vi "LIDAR V3.1 FPGA Main.vi"() -> ()   [LabVIEW 2013]
uses:
  Controls/FPGA Nain State.ctl
  <vilib>/Platform/TimedLoop/XDataNode/timing_clust.ctl
  <vilib>/Platform/TimedLoop/XDataNode/nitl_modes.ctl
  <vilib>/Platform/TimedLoop/XDataNode/wakeup.ctl
  Controls/Algorithm State.ctl
  <vilib>/rvi/Emulation/niFpgaSctlEmulationGetInTimedLoop.vi
  <vilib>/rvi/Emulation/niFpgaEmulationReportErrorSimple.vi
  <vilib>/rvi/Emulation/niFpgaGetClockAttributes.vi
  <vilib>/rvi/Emulation/niFpgaCriticalErrorInLSC.vi
  <vilib>/rvi/FIFO/Fifo_Resource/nirvififoEmulationReadFpgaImpl.vi
  <vilib>/rvi/DataTransferAndStorage/Container/Common/niFpgaContainerGetUniqueNameForEmu.vi
  <vilib>/rvi/FIFO/Fifo_Resource/nirvififoEmulationWriteFpgaImpl.vi
  <vilib>/rvi/interface/RandomDataEmulation/nirviRandomDataFPGAFIFO.vi
  <vilib>/rvi/interface/RandomDataEmulation/niFpgaRandomDataHandleErrors.vi
  <vilib>/rvi/eio/common/nirviEmuTemplateMethod_errors.vi
  <vilib>/rvi/Memory/Memory_Emulation/nirvimemoryFastEmulationFpgaImpl.vi
  <instcachedir>/0/nirvimemoryFastEmulationFpgaImpl_5FBAB50466BC4C939F684F8805638BFC.lvgen/nirvimemoryFastEmulationFpgaImpl_5FBAB50466BC4C939F684F8805638BFC_001.vi
  <vilib>/rvi/Memory/Memory_Emulation/nirvimemoryFastEmulation.vi
  <vilib>/rvi/Memory/Memory_Emulation/nirvimemoryEmulation.vi
  <vilib>/rvi/Emulation/niFpgaProcessEmulError.vi
  LIDAR V2 Globals.vi
  <instcachedir>/0/nirvimemoryFastEmulationFpgaImpl_5FBAB50466BC4C939F684F8805638BFC.lvgen/nirvimemoryFastEmulationFpgaImpl_5FBAB50466BC4C939F684F8805638BFC_005.vi
  <vilib>/Platform/TimedLoop/XDataNode/XDataNode.xnode
  <vilib>/rvi/DataTransferAndStorage/Container/XNode/niFpgaContainer.xnode
  <vilib>/rvi/FIFO/Fifo_Resource/nirvififoEmulationRead.vi
  <vilib>/rvi/FIFO/Fifo_Resource/nirvififoEmulationWrite.vi
  <vilib>/rvi/interface/RandomDataEmulation/nirviRandomDataFpgaReadWriteTemplate.vi
  <vilib>/eio/EIONode/EIONode.xnode
  <vilib>/Platform/TimedLoop/XDataNode/XDNodeRunTimeDep.lvlib
panel:
  in  "OutOFFValue":i16
  in  "OutONValue":i16=32767
  in  "FillDark":bool
  in  "DarkData":fxp<+/-,22,22>
  in  "DarkAdd":u32
  in  "SubstractDark":bool
  out "RawFifoWrite":bool
  out "AI Raw":u32
  out "LedIndex":u32
  in  "FillVga":bool
  in  "VgaData":i16
  in  "VgaAdd":u32
  in  "ScanMode":bool
  in  "FrameStartDisable":bool=TRUE
  out "MeanTimeouts":u16
  in  "MaxStartSample":u32
  in  "StreamToDMA":bool
  out "EndOfPulseGen":bool
  in  "SingleFrame":bool
  out "Port1":u8 format="%.0b"
  out "Port1Bit5":bool
  out "Port1Bit4":bool
  out "Port0":u8 format="%.0b"
  in  "PFI2":bool
  in  "PFI3":bool
  in  "WaitForPulseEndDelay":u8=3
  in  "ActiveLedIndexDeb":u16
  in  "LedScanDebEn":bool
  in  "NoOfLeds":u16=320
  out "LedAddress":u16
  in  "SamplingEnable":bool
  out "MainState":T1
  in  "PulseEndClck":u8=3
  in  "PulseWaitClck":u8=40
  out "SimOut":i16
  out "PulseIndex":i16
  in  "PulsePerLed":i16=199
  out "MemSel":bool
  out "ActiveLedIndex":u16
  in  "SampPerPulse":u16=100
  in  "PulseEnd":bool
  out "Timeouts":u16
  out "User Command Idle":bool
  out "User Command Status":u8
  out "User Error":bool
  out "Configured?":bool
  out "PLL Locked":bool
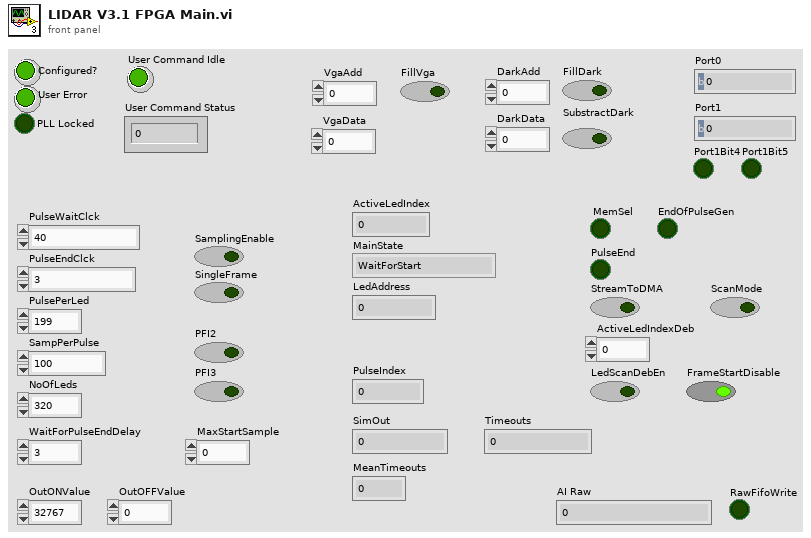
[diagram p1: front panel]
types:
  T1 = typedef "FPGA Nain State.ctl" = enum16{"WaitForStart", "SetProcParams", "SelectActiveLed", "WaitForPulseGenEnd", "ActivatePulse", "WaitForPulseEnd", "WaitForAlgoStart", "SingleCycleEnd"}
  T2 = typedef "XDNodeRunTimeDep.lvlib/timing_clust.ctl" = cluster{"Expected End [f-1]":u64, "Actual End [f-1]":u64, "Finished Late? [f-1]":bool, "Expected End [i-1]":u64, "Actual End [i-1]":u64, "Finished Late? [i-1]":bool, "Expected Start [i]":u64, "Actual Start [i]":u64, "Expected Start [f]":u64, "Actual Start [f]":u64, "Source Name":string, "Structure Name":string, "Period":i64, "Deadline":i64, "Offset":i64, "Start":i64, "Priority":i32, "Timeout":i32, "Mode":T3, "Wakeup Reason":T4, "Error":errorcluster, "Source Type":string, "Secondary Source Type":string, "Global End Time":u64, "Global Start Time":u64, "Frame Duration":u64, "Iteration Duration":u64, "Assigned CPU":i32, "I/O Scan Engine Mode":u32}
  T3 = typedef "XDNodeRunTimeDep.lvlib/nitl_modes.ctl" = enum32{"No Change", "Process missed periods, maintain original phase", "Discard missed periods, maintain original phase", "Process missed periods, ignore original phase", "Discard missed periods, ignore original phase"}
  T4 = typedef "XDNodeRunTimeDep.lvlib/wakeup.ctl" = enum32{"Normal", "Aborted", "Asynchronous wakeup", "Timing source error", "Timed loop error", "Timeout"}
  T5 = typedef "Algorithm State.ctl" = enum16{"WaitForStart", "GetNextSignalElement", "WaitForNextSignalElem", "MultWithSinc", "CalcMax"}
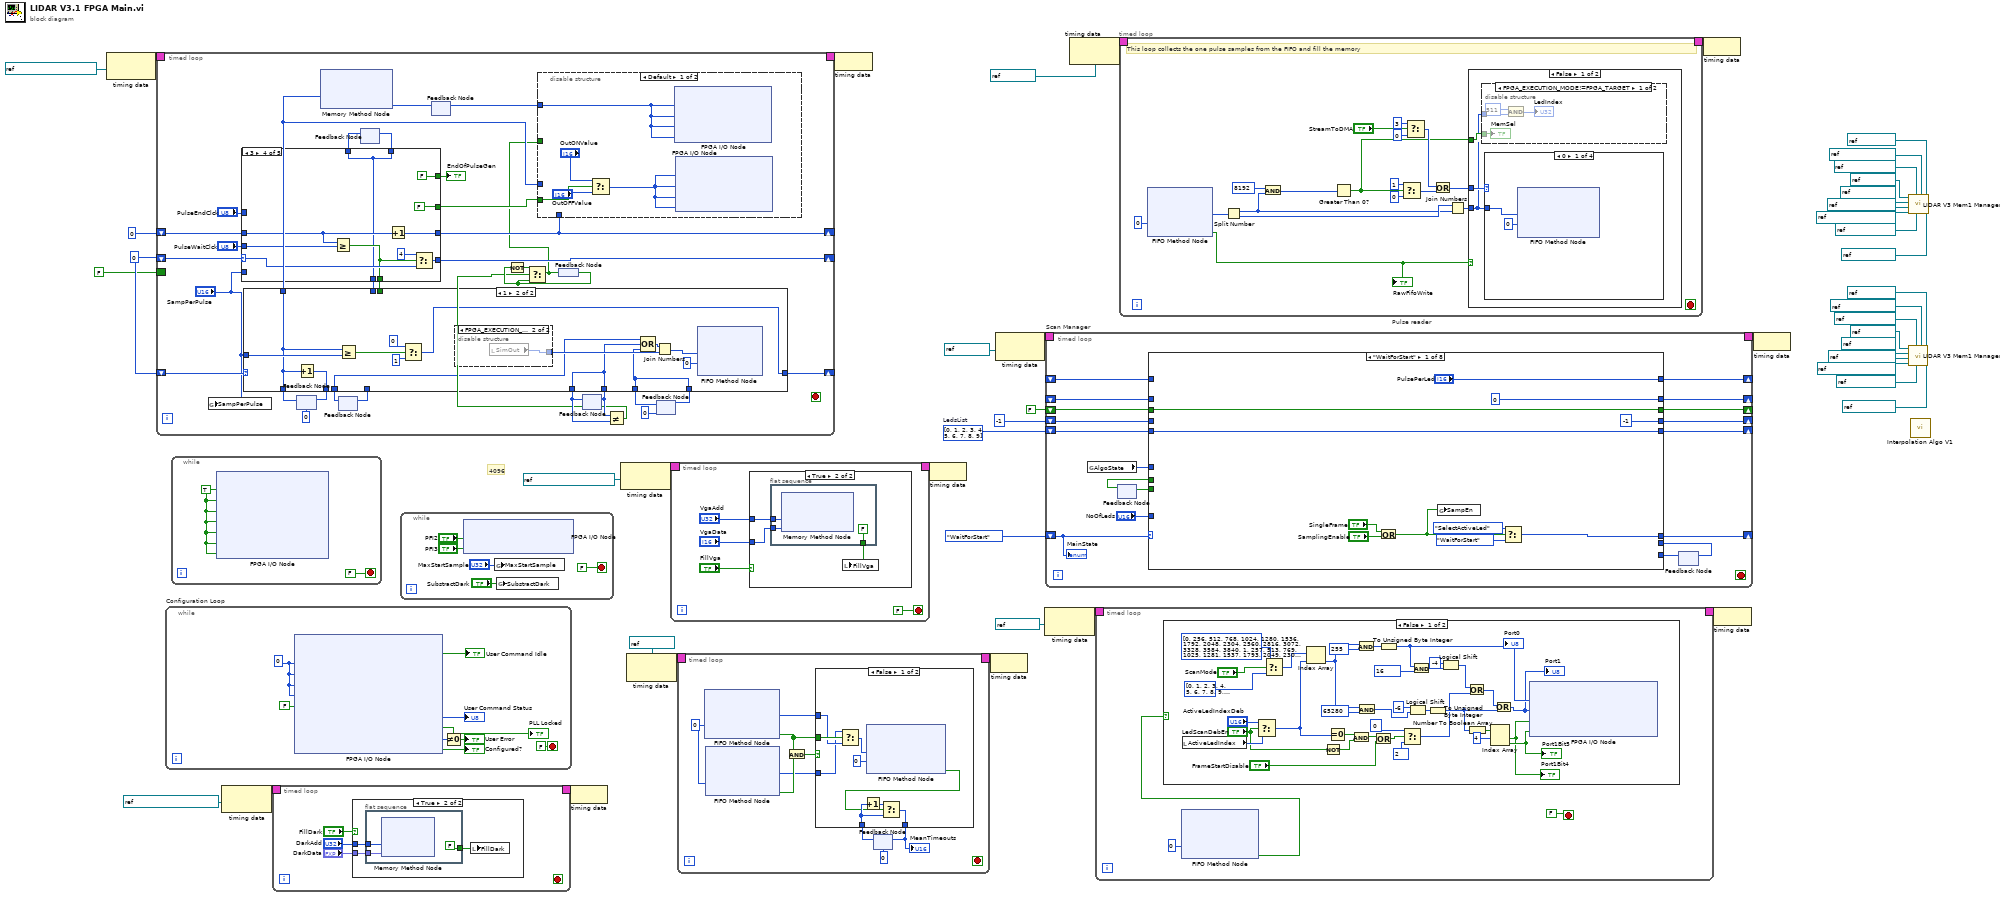
[diagram p0: block diagram]
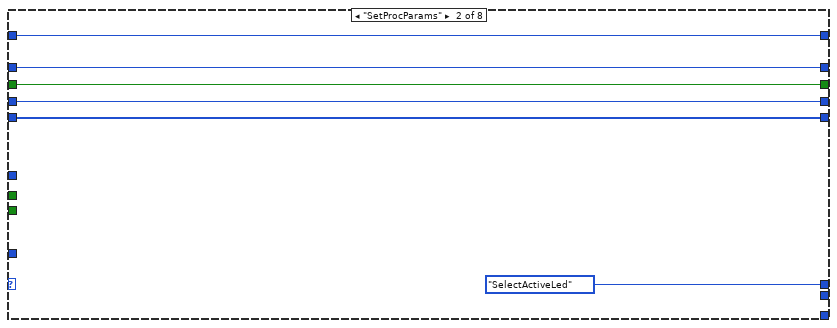
[diagram p6: hidden frame]
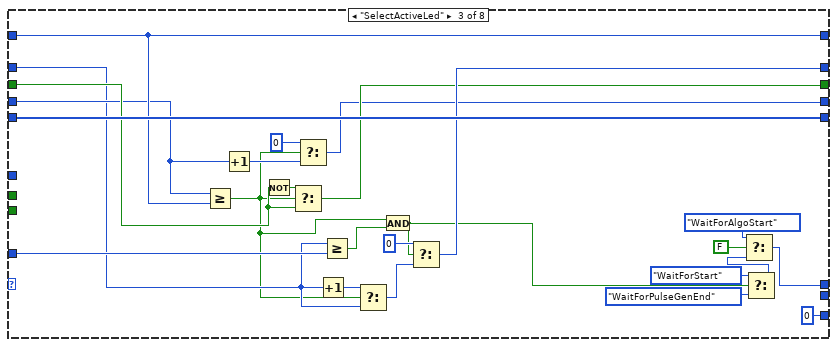
[diagram p7: hidden frame]
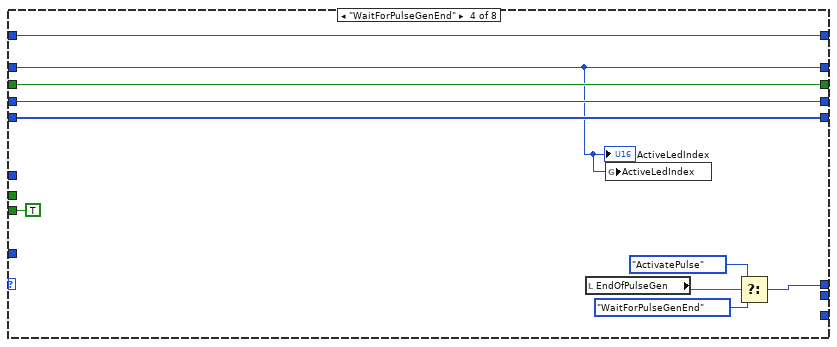
[diagram p8: hidden frame]
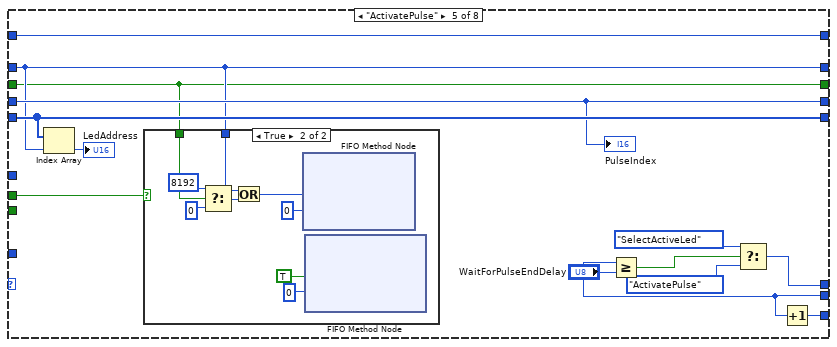
[diagram p9: hidden frame]
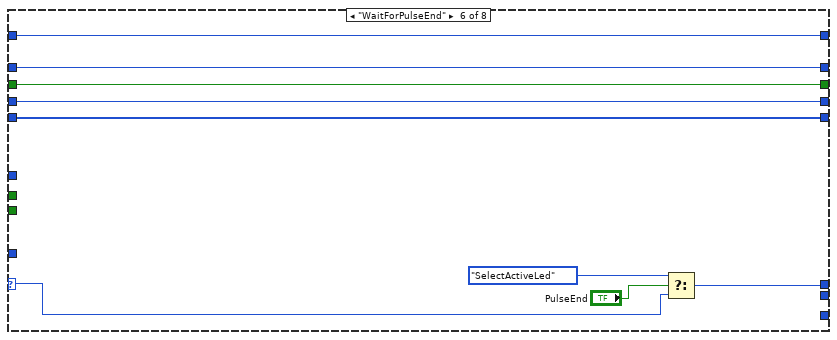
[diagram p11: hidden frame]
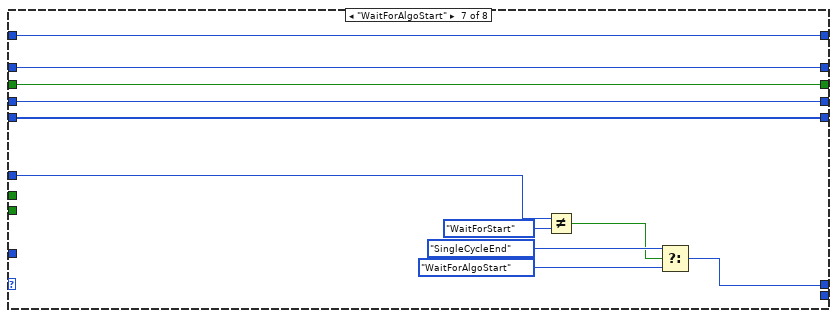
[diagram p12: hidden frame]
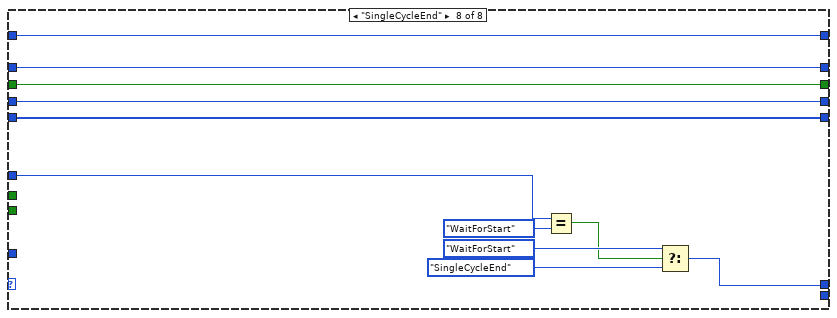
[diagram p13: hidden frame]
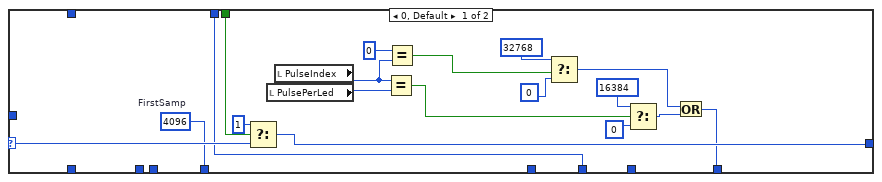
[diagram p14: hidden frame]
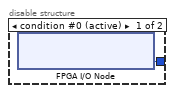
[diagram p15: hidden frame]
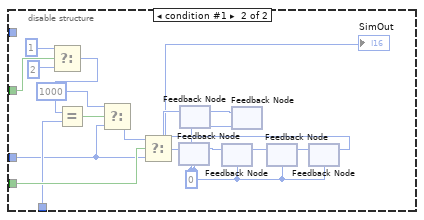
[diagram p16: hidden frame]
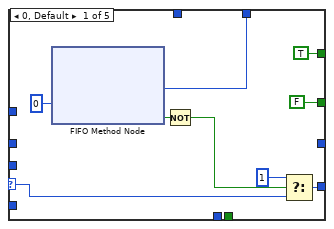
[diagram p17: hidden frame]
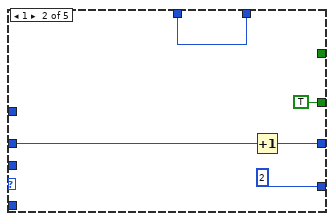
[diagram p18: hidden frame]
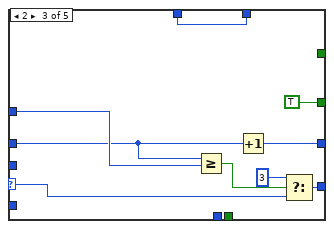
[diagram p19: hidden frame]
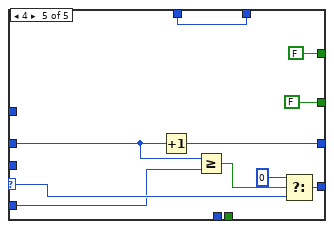
[diagram p20: hidden frame]
diagram:
  w35 = u16[] [0, 1, 2, 3, 4, 5, 6, 7, 8, 9]  # LedsList
  w30 = u8 0
  # "4096"
  n1 = node-c288(refnum<k21> "IO Module\\Data Clock" ("Source Name")) -> (w43:T2)
  n2 = timed-loop {
    timing: w43 -> [_]
    timing-out: [_] -> w42
    shift-right: [w77] -> _
    shift-left: w30 -> [w78]
    shift-right: [w75] -> _
    shift-left: u16 0 -> [w76]
    shift-right: [w67] -> _
    shift-left: w30 -> [w69]
    border: FALSE -> [_]
    stop <- _ stop-if-true
    n3 = global write "LIDAR V2 Globals.vi" "SampPerPulse"("SampPerPulse") -> ()
    n4 = feedback #1(u8 0) -> (w56:u8)
    n5 = feedback #2() -> (w58:u16)  [unwired: 1 in]
    n6 = feedback #3() -> (w65:u16)  [unwired: 1 in]
    n7 = case shown="3" w78 {
      selector: w78 -> [w137 _ w156 w166 w176]
      tunnel: [w143 u8 2 ("t") w157 w167 w177] -> w77
      tunnel: w76 -> [_ w147 w150 w162 w168]
      tunnel: [_ w148 w151 w163 w169] -> w75
      tunnel: [FALSE TRUE TRUE FALSE FALSE] -> w74
      tunnel: "PulseEndClck" -> [_ _ w153 _ _]
      tunnel: "PulseWaitClck" -> [_ _ _ w160 _]
      tunnel: "SampPerPulse" -> [_ _ _ _ w170]
      tunnel: [TRUE _ _ FALSE FALSE] -> w70
      tunnel: [_ _ _ w159 _] -> w68
      tunnel: [w135 w146 w149 w158 w171] -> w66
      tunnel: w65 -> [_ w146 w149 w158 w171]
      tunnel: [_ _ _ w158 _] -> w64
      frame 0, Default {
        n8 = xnode ("FIFO Method Node")("Timeout"=0) -> ("Element"=w135:u16, "Timed Out?"=w141:bool)  [unwired: 1 in, 1 out]
        n9 = Not(x=w141) -> (.not. x?=w139:bool)
        n10 = Select(t=u8 1, s=w139, f=w137) -> (s? t:f=w143:u8)
      }
      frame 1 {
        n11 = Increment(x=w147) -> (x+1=w148:u16)
      }
      frame 2 {
        n12 = Greater Or Equal?(x=w150, y=w153) -> (x >= y?=w152:bool)
        n13 = Increment(x=w150) -> (x+1=w151:u16)
        n14 = Select(t=u8 3, s=w152, f=w156) -> (s? t:f=w157:u8)
      }
      frame 3 {
        n15 = Greater Or Equal?(x=w162, y=w160) -> (x >= y?=w159:bool)
        n16 = Increment(x=w162) -> (x+1=w163:u16)
        n17 = Select(t=u8 4, s=w159, f=w166) -> (s? t:f=w167:u8)
      }
      frame 4 {
        n18 = Increment(x=w168) -> (x+1=w169:u16)
        n19 = Greater Or Equal?(x=w168, y=w170) -> (x >= y?=w173:bool)
        n20 = Select(t=u8 0, s=w173, f=w176) -> (s? t:f=w177:u8)
      }
    }
    "EndOfPulseGen" <- w70
    n21 = feedback-in #3(w66) -> ()
    n22 = feedback #4() -> (w54:i16)  [unwired: 1 in]
    n23 = feedback #5() -> (w51:bool)
    n24 = Not(x=w51) -> (.not. x?=w52:bool)
    n25 = feedback #6() -> (w48:u16)  [unwired: 1 in]
    n26 = feedback #7(u16 0) -> (w60:u16)
    n27 = case shown="1" w69 {
      selector: w69 -> [w95 _]
      tunnel: w68 -> [w96 _]
      tunnel: [w93 w101] -> w67
      tunnel: [w92 w100] -> w49
      tunnel: w64 -> [w92 _]
      tunnel: w48 -> [_ w100]
      tunnel: w56 -> [_ w97]
      tunnel: [_ w110] -> w62
      tunnel: "SampPerPulse" -> [_ w109]
      tunnel: [w82 w99] -> w61
      tunnel: w60 -> [_ w99]
      tunnel: [w81 _] -> w59
      tunnel: w58 -> [_ w98]
      tunnel: [_ w97] -> w53
      frame 0, Default {
        w81 = u16 4096  # FirstSamp
        n28 = Select(t=u8 1, s=w96, f=w95) -> (s? t:f=w93:u8)
        n29 = local read "PulsePerLed"() -> (w90:i16)
        n30 = local read "PulseIndex"() -> (w91:i16)
        n31 = Equal?(x=w91, y=w90) -> (x = y?=w87:bool)
        n32 = Equal?(x=i16 0, y=w91) -> (x = y?=w85:bool)
        n33 = Select(t=u16 32768 ("FirstIterration"), s=w85, f=u16 0 ("x")) -> (s? t:f=w83:u16)
        n34 = Select(t=u16 16384 ("LastIterration"), s=w87, f=u16 0 ("x")) -> (s? t:f=w84:u16)
        n35 = Or(x=w83, y=w84) -> (x .or. y?=w82:u16)
      }
      frame 1 {
        n36 = Increment(x=w97) -> (x+1=w110:u8)
        n37 = Greater Or Equal?(x=w97, y=w109) -> (x >= y?=w108:bool)
        n38 = Select(t=u8 0, s=w108, f=u8 1) -> (s? t:f=w101:u8)
        n39 = disable-structure shown="FPGA_EXECUTION_MODE!=FPGA_TARGET" {
          disable-tunnel: [w111 w112] -> w103
          frame condition #0 (active) {
            n40 = xnode "FPGA I/O Node"() -> ("IO Module\\AI 0 N"=w111:i16)  [unwired: 1 in, 1 out]
          }
          frame condition #1 {
            n41 = local read "SimOut"() -> (w112:i16)
          }
        }
        n42 = Compound Arithmetic op=OR(w98, w100, w99) -> (w105:u16)
        n43 = Join Numbers(hi=w105, lo=w103) -> ((hi.lo)=w104:u32)
        n44 = xnode ("FIFO Method Node")("Element"=w104, "Timeout"=0) -> ()  [unwired: 1 in, 2 out]
      }
    }
    n45 = feedback-in #1(w62) -> ()
    n46 = xnode ("Memory Method Node")("Address"=w53) -> ("Data"=w55:i16)  [unwired: 1 in, 1 out]
    n47 = feedback-in #2(w59) -> ()
    n48 = feedback-in #4(w55) -> ()
    n49 = feedback-in #6(w49) -> ()
    n50 = Not Equal?(x=w49, y=w48) -> (x != y?=w47:bool)
    n51 = Select(t=w52, s=w47, f=w51) -> (s? t:f=w50:bool)
    n52 = disable-structure shown="Default" {
      disable-tunnel: w74 -> [w115 w128]
      disable-tunnel: w75 -> [_ w127]
      disable-tunnel: w54 -> [w114 _]
      disable-tunnel: w53 -> [_ w123]
      disable-tunnel: w50 -> [_ w118]
      frame condition #0 (active) {
        n53 = Select(t="OutONValue", s=w115, f="OutOFFValue") -> (s? t:f=w116:i16)
        n54 = xnode "FPGA I/O Node"("IO Module\\AO 1 N"=w114, "IO Module\\AO 1 N-1"=w114, "IO Module\\AO 1 N-2"=w114, "IO Module\\AO 1 N-3"=w114) -> ()  [unwired: 4 in, 4 out]
        n55 = xnode "FPGA I/O Node"("IO Module\\AO 0 N-3"=w116, "IO Module\\AO 0 N-2"=w116, "IO Module\\AO 0 N-1"=w116, "IO Module\\AO 0 N"=w116) -> ()  [unwired: 4 in, 4 out]
      }
      frame condition #1 {
        w129 = i16 0 ("IO Module\\AO 0")
        n56 = Select(t=u16 1 ("x"), s=w118, f=u16 2 ("x")) -> (s? t:f=w119:u16)
        n57 = Equal?(x=w119, y=w127) -> (x = y?=w125:bool)
        n58 = Select(t=i16 1000 ("IO Module\\AO 0"), s=w125, f=w123) -> (s? t:f=w126:i16)
        n59 = Select(t=w126, s=w128, f=w123) -> (s? t:f=w122:i16)
        "SimOut" <- w122
        n60 = feedback-in #8(w122) -> ()
        n61 = feedback #8(w129) -> (w134:i16)
        n62 = feedback #9(w129) -> (w130:i16)
        n63 = feedback #10(w129) -> (w133:i16)
        n64 = feedback-in #10(w134) -> ()
        n65 = feedback #11(w129) -> ()  [unwired: 1 in]
        n66 = feedback-in #11(w130) -> ()
        n67 = feedback #12(w129) -> (w132:i16)
        n68 = feedback-in #12(w133) -> ()
        n69 = feedback #13(w129) -> (w131:i16)
        n70 = feedback-in #9(w131) -> ()
        n71 = feedback-in #13(w132) -> ()
      }
    }
    n72 = feedback-in #5(w50) -> ()
    n73 = feedback-in #7(w61) -> ()
  }
  n74 = while "Configuration Loop" {
    stop <- FALSE stop-if-true
    w181 = u8 0 ("SPI Device")
    n75 = xnode "FPGA I/O Node"("IO Module\\SPI Device"=w181, "IO Module\\User Command"=w181, "IO Module\\User Data 0"=w181, "IO Module\\User Data 1"=w181, "IO Module\\User Command Commit"=FALSE ("IO Module\\User Command Commit")) -> ("IO Module\\User Command Idle"=→"User Command Idle":bool, "IO Module\\User Command Status"=→"User Command Status":u8, "IO Module\\PLL Locked"=→"PLL Locked":bool, "IO Module\\User Error"=w185:u8, "IO Module\\Initialization Done"=→"Configured?":bool)  [unwired: 10 in, 10 out]
    n76 = Not Equal To 0?(x=w185) -> (x != 0?=→"User Error":bool)
  }
  n77 = while {
    stop <- FALSE stop-if-true
    w189 = TRUE ("IO Module\\DIO Port 0 WE")
    n78 = xnode "FPGA I/O Node"("IO Module\\DIO Port 0 WE"=w189, "IO Module\\DIO Port 1 WE"=w189, "IO Module\\PFI 0 WE"=w189, "IO Module\\PFI 1 WE"=w189, "IO Module\\PFI 2 WE"=w189, "IO Module\\PFI 3 WE"=w189, "IO Module\\AO Data Sync"=w189) -> ()  [unwired: 7 in, 7 out]
  }
  n79 = node-c288(refnum<k21> "40 MHz Onboard Clock" ("Source Name")) -> (w3:T2)
  n80 = timed-loop {
    timing: w3 -> [_]
    timing-out: [_] -> w2
    stop <- _ stop-if-true
    n81 = case shown="True" "FillDark" {
      tunnel: "DarkAdd" -> [_ w196]
      tunnel: "DarkData" -> [_ w195]
      frame False {
      }
      frame True {
        n82 = flat-sequence {
          tunnel: w196 -> [w199]
          tunnel: w195 -> [w198]
          tunnel: [FALSE] -> w194
          frame #0 {
            n83 = xnode ("Memory Method Node")("Address"=w199, "Data"=w198) -> ()  [unwired: 1 in, 1 out]
          }
        }
        n84 = local write "FillDark"(w194) -> ()
      }
    }
  }
  n85 = while {
    stop <- FALSE stop-if-true
    n86 = xnode "FPGA I/O Node"("IO Module\\PFI 2 Wr Data"="PFI2", "IO Module\\PFI 3 Wr Data"="PFI3") -> ()  [unwired: 2 in, 2 out]
    n87 = global write "LIDAR V2 Globals.vi" "MaxStartSample"("MaxStartSample") -> ()
    n88 = global write "LIDAR V2 Globals.vi" "SubstractDark"("SubstractDark") -> ()
  }
  n89 = node-c288(w2) -> ()
  n90 = node-c288(refnum<k21> "IO Module\\Data Clock" ("Source Name")) -> (w26:T2)
  n91 = node-c288(refnum<k21> "130MHz" ("Source Name")) -> (w29:T2)
  n92 = timed-loop {
    timing: w26 -> [_]
    timing-out: [_] -> w25
    stop <- FALSE stop-if-true
    n93 = case shown="True" "FillVga" {
      tunnel: "VgaAdd" -> [_ w213]
      tunnel: "VgaData" -> [_ w212]
      frame False {
      }
      frame True {
        n94 = flat-sequence {
          tunnel: w213 -> [w216]
          tunnel: w212 -> [w215]
          tunnel: [FALSE ("FillVga")] -> w211
          frame #0 {
            n95 = xnode ("Memory Method Node")("Address"=w216, "Data"=w215) -> ()  [unwired: 1 in, 1 out]
          }
        }
        n96 = local write "FillVga"(w211) -> ()
      }
    }
  }
  n97 = timed-loop {
    timing: w29 -> [_]
    timing-out: [_] -> w28
    stop <- _ stop-if-true
    w227 = 0 ("Timeout")
    n98 = xnode ("FIFO Method Node")("Timeout"=w227) -> ("Element"=w223:u32, "Timed Out?"=w224:bool)  [unwired: 1 in, 1 out]
    n99 = xnode ("FIFO Method Node")("Timeout"=w227) -> ("Element"=w222:u32, "Timed Out?"=w226:bool)  [unwired: 1 in, 1 out]
    n100 = And(x=w224, y=w226) -> (x .and. y?=w225:bool)
    n101 = feedback #14(u16 0) -> (w220:u16)
    n102 = case shown="False" w225 {
      tunnel: w224 -> [w235 _]
      tunnel: w223 -> [w234 _]
      tunnel: w222 -> [w233 _]
      tunnel: w220 -> [w230 w237]
      tunnel: [w231 w237] -> w219
      frame False {
        n103 = Select(t=w233, s=w235, f=w234) -> (s? t:f=w232:u32)
        n104 = Increment(x=w230) -> (x+1=w229:u16)
        n105 = xnode ("FIFO Method Node")("Element"=w232, "Timeout"=0) -> ("Timed Out?"=w228:bool)  [unwired: 1 in, 1 out]
        n106 = Select(t=w229, s=w228, f=w230) -> (s? t:f=w231:u16)
      }
      frame True {
      }
    }
    "MeanTimeouts" <- w219
    n107 = feedback-in #14(w219) -> ()
  }
  n108 = node-c288(w42) -> ()
  n109 = node-c288(w25) -> ()
  n110 = node-c288(w28) -> ()
  n111 = node-c288(refnum<k21> "130MHz" ("Source Name")) -> (w39:T2)
  n112 = node-c288(refnum<k21> "130MHz" ("Source Name")) -> (w33:T2)
  n113 = timed-loop "Scan Manager" {
    timing: w39 -> [_]
    timing-out: [_] -> w38
    shift-right: [w256] -> _
    shift-left: FPGA_Nain_State."WaitForStart" ("MainState") -> [w257]
    shift-right: [w255] -> _
    shift-left: _ -> [w254]
    shift-right: [w244] -> _
    shift-left: _ -> [w253]
    shift-right: [w248] -> _
    shift-left: FALSE -> [w252]
    shift-right: [w251] -> _
    shift-left: i16 -1 -> [w247]
    shift-right: [w249] -> _
    shift-left: w35 -> [w250]
    stop <- _ stop-if-true
    n114 = global read "LIDAR V2 Globals.vi" "AlgoState"() -> (w243:T5)
    n115 = feedback #15() -> (w245:bool)  [unwired: 1 in]
    n116 = feedback #16() -> (w240:u8)  [unwired: 1 in]
    n117 = case shown="\"WaitForStart\"" w257 {
      selector: w257 -> [_ _ _ _ _ w338 _ _]
      tunnel: [w266 FPGA_Nain_State."SelectActiveLed" ("MainState") w295 w302 w312 w337 w345 w356] -> w256
      tunnel: ["PulsePerLed" w271 w293 w309 w323 w341 w352 w363] -> w255
      tunnel: w254 -> [_ w271 w293 w309 w323 w341 w352 w363]
      tunnel: [u16 0 ("ActiveLedIndex") w270 w290 w301 w311 w340 w351 w362] -> w244
      tunnel: w253 -> [_ w270 w282 w301 w311 w340 w351 w362]
      tunnel: [w258 w269 w289 w308 w310 w339 w350 w361] -> w248
      tunnel: w252 -> [w258 w269 w292 w308 w310 w339 w350 w361]
      tunnel: [i16 -1 ("t") w273 w285 w307 w319 w335 w349 w360] -> w251
      tunnel: w247 -> [_ w273 w288 w307 w319 w335 w349 w360]
      tunnel: w250 -> [w265 w272 w299 w306 w320 w334 w348 w359]
      tunnel: [w265 w272 w299 w306 w320 w334 w348 w359] -> w249
      tunnel: [_ _ _ TRUE _ _ _ _] -> w246
      tunnel: w245 -> [_ _ _ _ w322 _ _ _]
      tunnel: w243 -> [_ _ _ _ _ _ w342 w354]
      tunnel: "NoOfLeds" -> [_ _ w284 _ _ _ _ _]
      tunnel: [_ _ u8 0 _ w318 _ _ _] -> w241
      tunnel: w240 -> [_ _ _ _ w317 _ _ _]
      frame "WaitForStart" {
        n118 = Or(x="SingleFrame", y="SamplingEnable") -> (x .or. y?=w260:bool)
        n119 = global write "LIDAR V2 Globals.vi" "SampEn"(w260) -> ()
        n120 = Select(t=FPGA_Nain_State."SelectActiveLed" ("MainState"), s=w260, f=FPGA_Nain_State."WaitForStart" ("MainState")) -> (s? t:f=w266:T1)
      }
      frame "SetProcParams" {
      }
      frame "SelectActiveLed" {
        n121 = Greater Or Equal?(x=w288, y=w293) -> (x >= y?=w277:bool)
        n122 = Increment(x=w288) -> (x+1=w287:i16)
        n123 = Not(x=w292) -> (.not. x?=w291:bool)
        n124 = Select(t=w291, s=w277, f=w292) -> (s? t:f=w289:bool)
        n125 = Select(t=i16 0, s=w277, f=w287) -> (s? t:f=w285:i16)
        n126 = Increment(x=w282) -> (x+1=w280:u16)
        n127 = Greater Or Equal?(x=w282, y=w284) -> (x >= y?=w278:bool)
        n128 = Select(t=w280, s=w277, f=w282) -> (s? t:f=w281:u16)
        n129 = And(x=w277, y=w278) -> (x .and. y?=w276:bool)
        n130 = Select(t=u16 0, s=w276, f=w281) -> (s? t:f=w290:u16)
        n131 = Select(t=FPGA_Nain_State."WaitForStart" ("MainState"), s=w276, f=FPGA_Nain_State."WaitForPulseGenEnd" ("MainState")) -> (s? t:f=w296:T1)
        n132 = Select(t=FPGA_Nain_State."WaitForAlgoStart" ("MainState"), s=FALSE, f=w296) -> (s? t:f=w295:T1)
      }
      frame "WaitForPulseGenEnd" {
        n133 = local read "EndOfPulseGen"() -> (w305:bool)
        n134 = global write "LIDAR V2 Globals.vi" "ActiveLedIndex"(w301) -> ()
        n135 = Select(t=FPGA_Nain_State."ActivatePulse" ("MainState"), s=w305, f=FPGA_Nain_State."WaitForPulseGenEnd" ("MainState")) -> (s? t:f=w302:T1)
        "ActiveLedIndex" <- w301
      }
      frame "ActivatePulse" {
        n136 = Index Array(array=w320, index=w311) -> (element=→"LedAddress":u16)
        n137 = case shown="True" w322 {
          tunnel: w311 -> [_ w329]
          tunnel: w310 -> [_ w326]
          frame False {
          }
          frame True {
            n138 = Select(t=u16 8192, s=w326, f=u16 0 ("t")) -> (s? t:f=w327:u16)
            n139 = Or(x=w329, y=w327) -> (x .or. y?=w328:u16)
            n140 = xnode ("FIFO Method Node")("Element"=w328, "Timeout"=0) -> ()  [unwired: 1 in, 2 out]
            n141 = xnode ("FIFO Method Node")("Element"=TRUE ("GenPulse"), "Timeout"=0) -> ()  [unwired: 1 in, 2 out]
          }
        }
        n142 = Greater Or Equal?(x=w317, y="WaitForPulseEndDelay") -> (x >= y?=w315:bool)
        n143 = Select(t=FPGA_Nain_State."SelectActiveLed" ("MainState"), s=w315, f=FPGA_Nain_State."ActivatePulse" ("MainState")) -> (s? t:f=w312:T1)
        n144 = Increment(x=w317) -> (x+1=w318:u8)
        "PulseIndex" <- w319
      }
      frame "WaitForPulseEnd" {
        n145 = Select(t=FPGA_Nain_State."SelectActiveLed", s="PulseEnd", f=w338) -> (s? t:f=w337:T1)
      }
      frame "WaitForAlgoStart" {
        n146 = Not Equal?(x=w342, y=Algorithm_State."WaitForStart") -> (x != y?=w343:bool)
        n147 = Select(t=FPGA_Nain_State."SingleCycleEnd", s=w343, f=FPGA_Nain_State."WaitForAlgoStart" ("MainState")) -> (s? t:f=w345:T1)
      }
      frame "SingleCycleEnd" {
        n148 = Equal?(x=w354, y=Algorithm_State."WaitForStart") -> (x = y?=w353:bool)
        n149 = Select(t=FPGA_Nain_State."WaitForStart", s=w353, f=FPGA_Nain_State."SingleCycleEnd" ("MainState")) -> (s? t:f=w356:T1)
      }
    }
    n150 = feedback-in #15(w246) -> ()
    n151 = feedback-in #16(w241) -> ()
    "MainState" <- w257
  }
  n152 = node-c288(refnum<k21> "130MHz" ("Source Name")) -> (w46:T2)
  n153 = timed-loop {
    timing: w33 -> [_]
    timing-out: [_] -> w32
    stop <- FALSE stop-if-true
    n154 = xnode ("FIFO Method Node")("Timeout"=0) -> ("Timed Out?"=w366:bool)  [unwired: 1 in, 2 out]
    n155 = case shown="False" w366 {
      frame False {
        n156 = local read "ActiveLedIndex"() -> (w399:u16)
        n157 = Select(t="ActiveLedIndexDeb", s="LedScanDebEn", f=w399) -> (s? t:f=w384:u16)
        n158 = Select(t=u16[] [0, 256, 512, 768, 1024, 1280, 1536, 1792, 2048, 2304, 2560, 2816, 3072, 3328, 3584, 3840, 1, 257, 513, 769, 1025, 1281, 1537, 1793, 2049, 2305, 2561, 2817, 3073, 3329, 3585, 3841, 2, 258, 514, 770, 1026, 1282, 1538, 1794, 2050, 2306, 2562, 2818, 3074, 3330, 3586, 3842, 3, 259, 515, 771, 1027, 1283, 1539, 1795, 2051, 2307, 2563, 2819, 3075, 3331, 3587, 3843, 4, 260, 516, 772, 1028, 1284, 1540, 1796, 2052, 2308, 2564, 2820, 3076, 3332, 3588, 3844, 5, 261, 517, 773, 1029, 1285, 1541, 1797, 2053, 2309, 2565, 2821, 3077, 3333, 3589, 3845, 6, 262, 518, 774, 1030, 1286, 1542, 1798, 2054, 2310, 2566, 2822, 3078, 3334, 3590, 3846, 7, 263, 519, 775, 1031, 1287, 1543, 1799, 2055, 2311, 2567, 2823, 3079, 3335, 3591, 3847, 8, 264, 520, 776, 1032, 1288, 1544, 1800, 2056, 2312, 2568, 2824, 3080, 3336, 3592, 3848, 9, 265, 521, 777, 1033, 1289, 1545, 1801, 2057, 2313, 2569, 2825, 3081, 3337, 3593, 3849, 10, 266, 522, 778, 1034, 1290, 1546, 1802, 2058, 2314, 2570, 2826, 3082, 3338, 3594, 3850, 11, 267, 523, 779, 1035, 1291, 1547, 1803, 2059, 2315, 2571, 2827, 3083, 3339, 3595, 3851, 12, 268, 524, 780, 1036, 1292, 1548, 1804, 2060, 2316, 2572, 2828, 3084, 3340, 3596, 3852, 13, 269, 525, 781, 1037, 1293, 1549, 1805, 2061, 2317, 2573, 2829, 3085, 3341, 3597, 3853, 14, 270, 526, 782, 1038, 1294, 1550, 1806, 2062, 2318, 2574, 2830, 3086, 3342, 3598, 3854, 15, 271, 527, 783, 1039, 1295, 1551, 1807, 2063, 2319, 2575, 2831, 3087, 3343, 3599, 3855, 16, 272, 528, 784, 1040, 1296, 1552, 1808, 2064, 2320, 2576, 2832, 3088, 3344, 3600, 3856, 17, 273, 529, 785, 1041, 1297, 1553, 1809, 2065, 2321, 2577, 2833, 3089, 3345, 3601, 3857, 18, 274, 530, 786, 1042, 1298, 1554, 1810, 2066, 2322, 2578, 2834, 3090, 3346, 3602, 3858, 19, 275, 531, 787, 1043, 1299, 1555, 1811, 2067, 2323, 2579, 2835, 3091, 3347, 3603, 3859] ("Array"), s="ScanMode", f=u16[] [0, 1, 2, 3, 4, 5, 6, 7, 8, 9, 10, 11, 12, 13, 14, 15, 16, 17, 18, 19, 256, 257, 258, 259, 260, 261, 262, 263, 264, 265, 266, 267, 268, 269, 270, 271, 272, 273, 274, 275, 512, 513, 514, 515, 516, 517, 518, 519, 520, 521, 522, 523, 524, 525, 526, 527, 528, 529, 530, 531, 768, 769, 770, 771, 772, 773, 774, 775, 776, 777, 778, 779, 780, 781, 782, 783, 784, 785, 786, 787, 1024, 1025, 1026, 1027, 1028, 1029, 1030, 1031, 1032, 1033, 1034, 1035, 1036, 1037, 1038, 1039, 1040, 1041, 1042, 1043, 1280, 1281, 1282, 1283, 1284, 1285, 1286, 1287, 1288, 1289, 1290, 1291, 1292, 1293, 1294, 1295, 1296, 1297, 1298, 1299, 1536, 1537, 1538, 1539, 1540, 1541, 1542, 1543, 1544, 1545, 1546, 1547, 1548, 1549, 1550, 1551, 1552, 1553, 1554, 1555, 1792, 1793, 1794, 1795, 1796, 1797, 1798, 1799, 1800, 1801, 1802, 1803, 1804, 1805, 1806, 1807, 1808, 1809, 1810, 1811, 2048, 2049, 2050, 2051, 2052, 2053, 2054, 2055, 2056, 2057, 2058, 2059, 2060, 2061, 2062, 2063, 2064, 2065, 2066, 2067, 2304, 2305, 2306, 2307, 2308, 2309, 2310, 2311, 2312, 2313, 2314, 2315, 2316, 2317, 2318, 2319, 2320, 2321, 2322, 2323, 2560, 2561, 2562, 2563, 2564, 2565, 2566, 2567, 2568, 2569, 2570, 2571, 2572, 2573, 2574, 2575, 2576, 2577, 2578, 2579, 2816, 2817, 2818, 2819, 2820, 2821, 2822, 2823, 2824, 2825, 2826, 2827, 2828, 2829, 2830, 2831, 2832, 2833, 2834, 2835, 3072, 3073, 3074, 3075, 3076, 3077, 3078, 3079, 3080, 3081, 3082, 3083, 3084, 3085, 3086, 3087, 3088, 3089, 3090, 3091, 3328, 3329, 3330, 3331, 3332, 3333, 3334, 3335, 3336, 3337, 3338, 3339, 3340, 3341, 3342, 3343, 3344, 3345, 3346, 3347, 3584, 3585, 3586, 3587, 3588, 3589, 3590, 3591, 3592, 3593, 3594, 3595, 3596, 3597, 3598, 3599, 3600, 3601, 3602, 3603, 3840, 3841, 3842, 3843, 3844, 3845, 3846, 3847, 3848, 3849, 3850, 3851, 3852, 3853, 3854, 3855, 3856, 3857, 3858, 3859] ("Array")) -> (s? t:f=w370:u16[])
        n159 = Index Array(array=w370, index=w384) -> (element=w396:u16)
        n160 = Not(x="LedScanDebEn") -> (.not. x?=w381:bool)
        n161 = Equal To 0?(x=w384) -> (x = 0?=w383:bool)
        n162 = And(x=w383, y=w381) -> (x .and. y?=w379:bool)
        n163 = And(x=w396, y=u16 255) -> (x .and. y?=w394:u16)
        n164 = And(x=w396, y=u16 65280) -> (x .and. y?=w393:u16)
        n165 = Or(x=w379, y="FrameStartDisable") -> (x .or. y?=w374:bool)
        n166 = To Unsigned Byte Integer(number=w394) -> (unsigned 8bit integer=w390:u8)
        "Port0" <- w390
        n167 = Select(t=u8 0, s=w374, f=u8 2) -> (s? t:f=w376:u8)
        n168 = Logical Shift(y=i16 -6, x=w393) -> (x << y=w392:u16)
        n169 = And(x=w390, y=u8 16) -> (x .and. y?=w389:u8)
        n170 = To Unsigned Byte Integer(number=w392) -> (unsigned 8bit integer=w386:u8)
        n171 = Logical Shift(y=i16 -4, x=w389) -> (x << y=w380:u8)
        n172 = Or(x=w380, y=w376) -> (x .or. y?=w375:u8)
        n173 = Number To Boolean Array(number=w386) -> (Boolean array=w403:bool[])
        n174 = Index Array(array=w403, index #1=4 ("index")) -> (element #1=w387:bool, element #2=w401:bool)  [unwired: 1 in]
        "Port1Bit4" <- w387
        "Port1Bit5" <- w401
        n175 = Or(x=w375, y=w386) -> (x .or. y?=w385:u8)
        "Port1" <- w385
        n176 = xnode "FPGA I/O Node"("IO Module\\DIO Port 0 Wr Data"=w390, "IO Module\\DIO Port 1 Wr Data"=w385, "IO Module\\PFI 0 Wr Data"=w387, "IO Module\\PFI 1 Wr Data"=w401) -> ()  [unwired: 4 in, 4 out]
      }
      frame True {
      }
    }
  }
  n177 = timed-loop "Pulse reader" {
    timing: w46 -> [_]
    timing-out: [_] -> w45
    stop <- _ stop-if-true
    # "This loop collects the one pulse samples from the FIFO and fill the memory"
    n178 = xnode ("FIFO Method Node")("Timeout"=0) -> ("Element"=w421:u32, "Timed Out?"=w408:bool)  [unwired: 1 in, 1 out]
    "RawFifoWrite" <- w408
    n179 = Split Number(x=w421) -> (hi(x)=w406:u16, lo(x)=w410:u16)
    n180 = And(x=u16 8192, y=w406) -> (x .and. y?=w413:u16)
    n181 = Greater Than 0?(x=w413) -> (x > 0?=w407:bool)
    n182 = Select(t=i16 1, s=w407, f=i16 0) -> (s? t:f=w417:i16)
    n183 = Select(t=i16 3, s="StreamToDMA", f=i16 0) -> (s? t:f=w416:i16)
    n184 = Or(x=w416, y=w417) -> (x .or. y?=w412:i16)
    n185 = Join Numbers(hi=w410, lo=w406) -> ((hi.lo)=w409:u32)
    n186 = case shown="False" w408 {
      tunnel: w412 -> [w425 _]
      tunnel: w409 -> [w423 _]
      tunnel: w407 -> [w424 _]
      frame False {
        n187 = disable-structure shown="FPGA_EXECUTION_MODE!=FPGA_TARGET" {
          disable-tunnel: w424 -> [w429 _]
          disable-tunnel: w423 -> [w428 _]
          frame condition #0 {
            n188 = And(x=u32 511, y=w428) -> (x .and. y?=→"LedIndex":u32)
            "MemSel" <- w429
          }
          frame condition #1 (active) {
          }
        }
        n189 = case shown="0" w425 {
          tunnel: w423 -> [w430 w432 _ w434]
          frame 0 {
            n190 = xnode ("FIFO Method Node")("Element"=w430, "Timeout"=0) -> ()  [unwired: 1 in, 2 out]
          }
          frame 1 {
            n191 = xnode ("FIFO Method Node")("Element"=w432, "Timeout"=0) -> ()  [unwired: 1 in, 2 out]
          }
          frame Default {
          }
          frame 3 {
            n192 = disable-structure shown="Default" {
              disable-tunnel: w434 -> [w435 w442]
              frame condition #0 (active) {
                n193 = xnode ("FIFO Method Node")("Element"=w435, "Timeout"=0) -> ("Timed Out?"=w437:bool)  [unwired: 1 in, 1 out]
                n194 = feedback #17(u16 0) -> (w440:u16)
                n195 = Increment(x=w440) -> (x+1=w441:u16)
                n196 = Select(t=w441, s=w437, f=w440) -> (s? t:f=w439:u16)
                "Timeouts" <- w439
                n197 = feedback-in #17(w439) -> ()
              }
              frame condition #1 {
                "AI Raw" <- w442
              }
            }
          }
        }
      }
      frame True {
      }
    }
  }
  n198 = node-c288(w45) -> ()
  n199 = node-c288(w32) -> ()
  n200 = node-c288(w38) -> ()
  n201 = call "LIDAR V3 Mem1 Manager.vi"("MeanFIFO"=refnum<k21> "MeanVals1", "StartAlgo"=refnum<k21> "StartAlg1", "MemRequest"=refnum<k21> "MemRequest1", "SignalMem"=refnum<k21> "SignalMem1", "MemDataAi"=refnum<k21> "MemDataAi1", "MemRequestDeb"=refnum<k21> "MemRequestDeb1", "MemDataDeb"=refnum<k21> "MemDataDeb1", "MemData"=refnum<k21> "MemData1", "Source Clk"=refnum<k21> "130MHz" ("Source Name")) -> ()  [unwired: 3 in]
  n202 = call "LIDAR V3 Mem1 Manager.vi"("MeanFIFO"=refnum<k21> "MeanVals2", "StartAlgo"=refnum<k21> "StartAlg2", "MemRequest"=refnum<k21> "MemRequest2", "SignalMem"=refnum<k21> "SignalMem2", "MemDataAi"=refnum<k21> "MemDataAi2", "MemRequestDeb"=refnum<k21> "MemRequestDeb2", "MemDataDeb"=refnum<k21> "MemDataDeb2", "MemData"=refnum<k21> "MemData2", "Source Clk"=refnum<k21> "130MHz" ("Source Name")) -> ()  [unwired: 3 in]
  n203 = call "Interpolation Algo V1.vi"() -> ()  [unwired: 10 in, 2 out]
